vi "arcade.vi"(9 "Y-Axis":dbl, 11 "X-Axis":dbl) -> (1 "Left":dbl, 3 "Right":dbl)   [LabVIEW 2016]
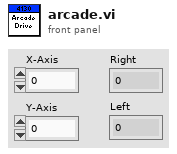
[diagram p1: front panel]
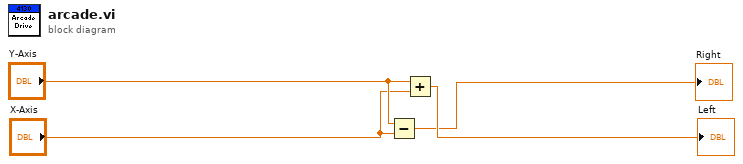
[diagram p0: block diagram]
diagram:
  n1 = Subtract(x="Y-Axis", y="X-Axis") -> (x-y=→"Right":dbl)
  n2 = Add(x="Y-Axis", y="X-Axis") -> (x+y=→"Left":dbl)
